vi "Connection State.vi"(8 "error in (no error)":errorcluster, 11 "VolatusAPI in":refnum<class "VolatusAPI.lvclass">) -> (0 "error out":errorcluster, 2 "Connected Status":T1=enum."Connected", 3 "VolatusAPI out":refnum<class "VolatusAPI.lvclass">)   [LabVIEW 2020, in "Volatus.lvlib" / "VolatusAPI.lvclass"]
uses:
  VolatusAPI.lvclass
  VolatusAPI.lvclass/VolatusAPI.ctl
  lv-vecto/Vecto/TCPMessageService/TCPMessageAPI.lvclass
  lv-vecto/Vecto/Connected Status.ctl
  lv-vecto/Vecto/Vecto.lvlib
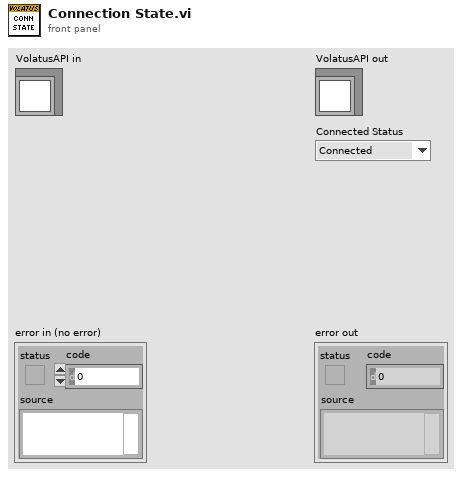
[diagram p1: front panel]
types:
  T1 = typedef "Vecto.lvlib/Connected Status.ctl" = enum16{"Disconnected", "Connected", "Bad Config", "Not Allowed", "Server"}
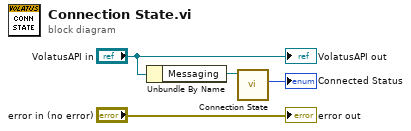
[diagram p0: block diagram]
diagram:
  n1 = Unbundle By Name("VolatusAPI in") -> ("Messaging"=w2:refnum<class "TCPMessageAPI.lvclass">)
  n2 = call "Connection State.vi"("TCPMessageAPI in"=w2) -> ("Connected"=→"Connected Status":T1)  [unwired: 8 in, 2 out]
  "error out" <- "error in (no error)"
  "VolatusAPI out" <- "VolatusAPI in"
